vi "ni579x Configure Attenuation.vi"(0 "Register Bus":T1, 1 "scope":string(combo)="rx/atten1", 5 "attenuation [dB]":dbl format="%#_6p", 11 "Error In":errorcluster) -> (4 "Register Bus (out)":T1, 6 "coerced attenuation [dB]":dbl format="%#_6p", 15 "Error Out":errorcluster)   [LabVIEW 2015, in "ni579x Config v2 Host.lvlib"]
uses:
  <instrlib>/ni579x/Config/v2/Host/ni579x Config v2 Host.lvlib
  <instrlib>/_niInstr/Register Bus/v0/Host/Public/Register Bus Session.ctl
  <instrlib>/_niInstr/Register Bus/v0/Host/Private/Session Data.ctl
  <instrlib>/_niInstr/Register Bus/v0/Host/niInstr Register Bus v0 Host.lvlib
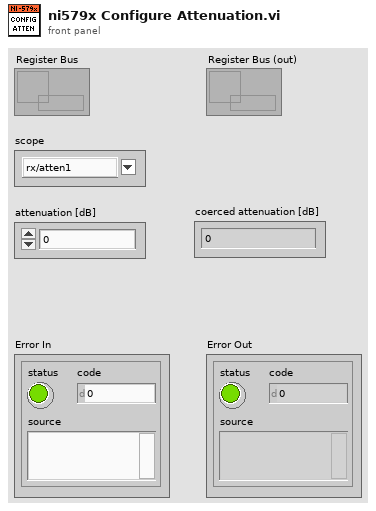
[diagram p1: front panel]
types:
  T1 = typedef "niInstr Register Bus v0 Host.lvlib/Register Bus Session.ctl" = refnum<queue>
  T2 = typedef "ni579x Config v2 Shared.lvlib/ni579x User Command.ctl" = cluster{"User Data 0":u8, "User Data 1":u8, "User Command ID":T3}
  T3 = typedef "ni579x Config v2 Shared.lvlib/ni579x User Command ID.ctl" = u8
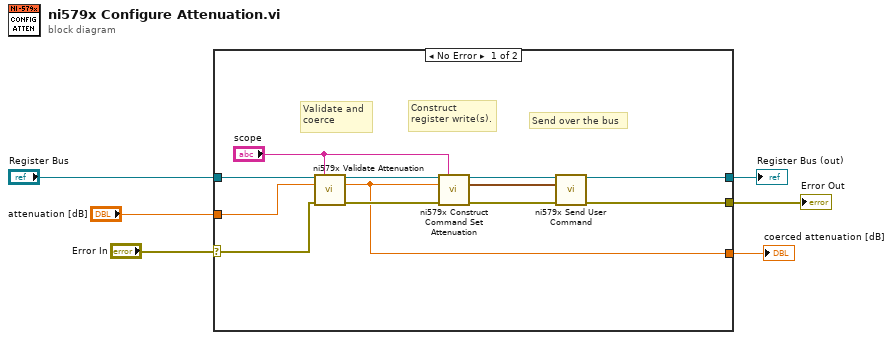
[diagram p0: block diagram]
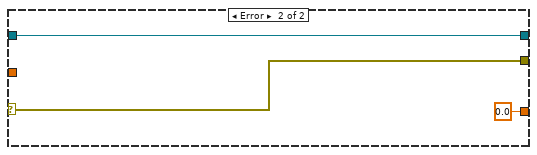
[diagram p2: hidden frame]
diagram:
  n1 = case shown="No Error" "Error In" {
    selector: "Error In" -> [w16 w21]
    tunnel: [w9 w21] -> w5
    tunnel: "Register Bus" -> [w18 w20]
    tunnel: "attenuation [dB]" -> [w17 _]
    tunnel: [w10 w20] -> w2
    tunnel: [w8 0.0 ("coerced attenuation [dB]")] -> w1
    frame No Error {
      # "Send over the bus"
      # "Construct\nregister write(s)."
      # "Validate and \ncoerce"
      n2 = call <instrlib>:"ni579x Validate Attenuation.vi"("Register Bus"=w18, "scope"="scope", "attenuation [dB]"=w17, "Error In"=w16) -> ("Register Bus (out)"=w14:T1, "coerced attenuation [dB]"=w8:dbl, "Error Out"=w15:errorcluster)  [unwired: 9 in]
      n3 = call <instrlib>:"ni579x Construct Command Set Attenuation.vi"("Register Bus"=w14, "scope"="scope", "attenuation [dB]"=w8, "Error In"=w15) -> ("Register Bus (out)"=w12:T1, "User Command"=w7:T2, "Error Out"=w11:errorcluster)  [unwired: 9 in]
      n4 = call <instrlib>:"ni579x Send User Command.vi"("Register Bus"=w12, "User Command"=w7, "Error In"=w11) -> ("Register Bus (out)"=w10:T1, "Error Out"=w9:errorcluster)  [unwired: 8 in, 3 out]
    }
    frame Error {
    }
  }
  "Register Bus (out)" <- w2
  "Error Out" <- w5
  "coerced attenuation [dB]" <- w1
